vi "get_addressee.vi"(0 "MoAgSy_Message in":refnum<class "MoAgSy_Message.lvclass">, 5 "error in (no error)":errorcluster) -> (14 "MoAgSy_Message out":refnum<class "MoAgSy_Message.lvclass">, 17 "addressee":string, 19 "error out":errorcluster)   [LabVIEW 2009, in "MoAgSy.lvlib" / "MoAgSy_Message.lvclass"]
uses:
  MoAgSy_Message.lvclass
  MoAgSy_Message.lvclass/MoAgSy_Message.ctl
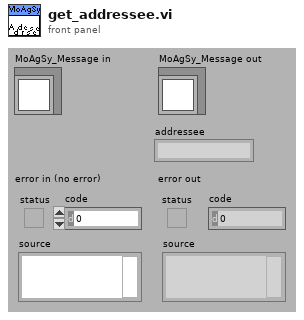
[diagram p1: front panel]
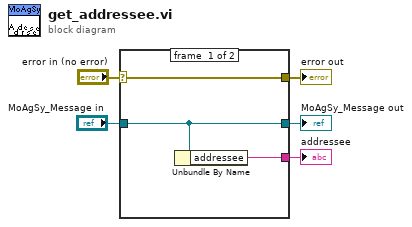
[diagram p0: block diagram]
diagram:
  n1 = case shown="No Error" "error in (no error)" {
    selector: "error in (no error)" -> [w8 w10]
    tunnel: [w8 w10] -> w4
    tunnel: [w7 w9] -> w2
    tunnel: "MoAgSy_Message in" -> [w7 w9]
    tunnel: [w6 _] -> w1
    frame #0 {
      n2 = Unbundle By Name(w7) -> ("addressee"=w6:string)
    }
    frame #1 {
    }
  }
  "error out" <- w4
  "MoAgSy_Message out" <- w2
  "addressee" <- w1
